vi "Error Message Handler.vi"(8 "Error In":errorcluster) -> (0 "Error Out":errorcluster, 3 "T button?":bool)   [LabVIEW 2014]
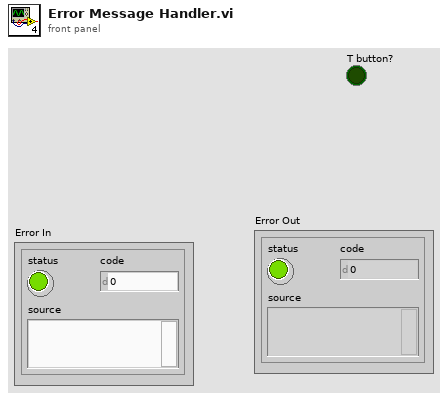
[diagram p1: front panel]
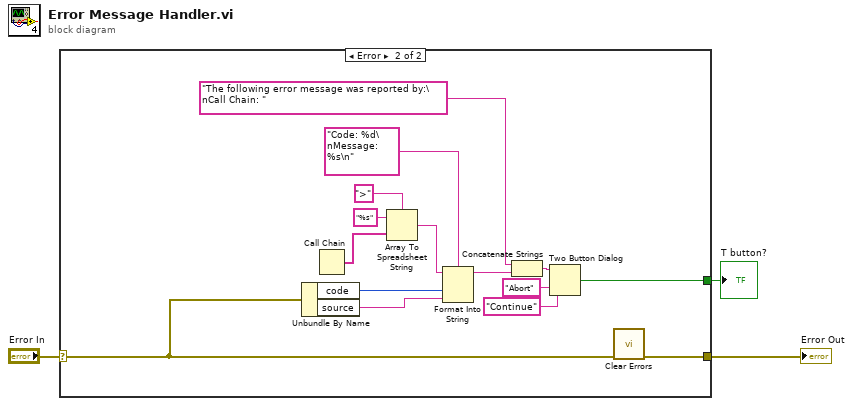
[diagram p0: block diagram]
diagram:
  n1 = case shown="Error" "Error In" {
    selector: "Error In" -> [w4 w17]
    tunnel: [w4 w19] -> w2
    tunnel: [_ w7] -> w1
    frame No Error {
    }
    frame Error {
      n2 = Unbundle By Name(w17) -> ("code"=w16:i32, "source"=w15:string)
      n3 = Call Chain() -> (call chain=w18:string[])
      n4 = Array To Spreadsheet String(delimiter (Tab)=">", array=w18, 3:"%s" ("format string")) -> (spreadsheet string=w13:string)
      n5 = Format Into String(format string="Code: %d\nMessage: %s\n", initial string=w13, w16, w15) -> (resulting string=w12:string)  [unwired: 1 in, 1 out]
      n6 = Concatenate Strings("The following error message was reported by:\nCall Chain: ", w12) -> (w9:string)
      n7 = Two Button Dialog(message=w9, 1:"Continue" ("F button name (\"Cancel\")"), 2:"Abort" ("T button name (\"OK\")")) -> (T button?=w7:bool)
      n8 = call <vilib>:"Clear Errors.vi"("error in (no error)"=w17) -> ("error out"=w19:errorcluster)  [unwired: 5 in, 1 out]
    }
  }
  "Error Out" <- w2
  "T button?" <- w1
